vi "TmpVi.vi"   [LabVIEW 2011]
uses:
  <vilib>/Utility/NIReport.llb/NI_report.lvclass
  <vilib>/addons/_office/NI_ReportGenerationToolkit.lvlib
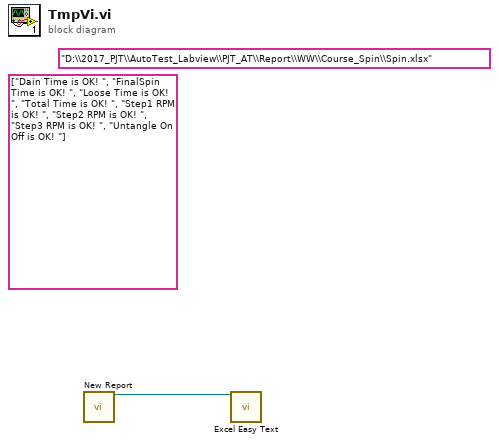
[diagram p0: block diagram]
diagram:
  (unwired) "D:\\2017_PJT\\AutoTest_Labview\\PJT_AT\\Report\\WW\\Course_Spin\\Spin.xlsx"
  (unwired) string[] ["Dain Time is OK! ", "FinalSpin Time is OK! ", "Loose Time is OK! ", "Total Time is OK! ", "Step1 RPM is OK! ", "Step2 RPM is OK! ", "Step3 RPM is OK! ", "Untangle On Off is OK! "] ("strArrayError")
  n1 = call <vilib>:"New Report.vi"() -> ("report out"=w1:refnum<class "NI_report.lvclass">)  [unwired: 14 in, 1 out]
  n2 = call <vilib>:"Excel Easy Text.vi"("report in"=w1) -> ()  [unwired: 10 in, 5 out]
